vi "Hardware-DIScope.vi"(11 "DSI Reference":refnum<class "DCM-DSI.lvclass">) -> ()   [LabVIEW 2016, in "DSI-RT.lvlib"]
uses:
  DSI-RT.lvlib
  Classes/DCM-DSI/DCM-DSI.lvclass
  <vilib>/Powertrain Controls/Device Drivers/DCM/Rev0/RT/DI - ADC Select.ctl
  <vilib>/Powertrain Controls/Device Drivers/DCM/Rev0/FPGA/DI - ADC Signals.ctl
  <vilib>/Powertrain Controls/Device Drivers/DCM/Rev0/RT/DCM - RT.lvclass/DCM - RT.ctl
  <vilib>/Powertrain Controls/Device Drivers/DCM/Rev0/RT/Read Stop Target.vi
  Classes/DCM-DSI/Read DCM Ref.vi
  Classes/DCM-DSI/Write DI Scope dt.vi
  Classes/DCM-DSI/Write DI Scope Data.vi
  <vilib>/Powertrain Controls/Device Drivers/DCM/Rev0/RT/DCM - RT.lvclass
  <vilib>/addons/Software Calibration Management/xSCM/CalPoint.xnode
  <vilib>/Powertrain Controls/Device Drivers/DCM/DI/RT/DCM - RT - DI.lvlib
  <vilib>/Powertrain Controls/Device Drivers/DCM/Rev0/FPGA/DCM - FPGA.lvlib
  <vilib>/addons/Software Calibration Management/xSCM/ni_scm.dll
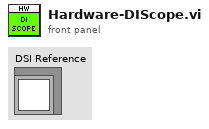
[diagram p1: front panel]
types:
  T1 = typedef "DCM - RT.lvclass/DI - ADC Select.ctl" = cluster{"DI ADC 1":T2, "DI ADC 2":T2, "DI ADC 3":T2, "DI ADC 4":T2}
  T2 = typedef "DCM - FPGA.lvlib/DI - ADC Signals.ctl" = enum8{"I LS A1/A5", "I LS A2/A6", "I LS A3/A7", "I LS A4", "I LS A8/PumpA", "V PZ A1", "V PZ A2", "V PZ A3", "V PZ A4", "V S A1", "V S A2", "V S A3", "V S A4", "V S A5", "V S A6", "V S A7", "V S A8", "V Pump A", "V Secondary A1A2", "V Secondary A3A4", "V Ext HV A", "------------------------ ", "I LS B1/B5", "I LS B2/B6", "I LS B3/B7", "I LS B4", "I LS B8/PumpB", "V PZ B1", "V PZ B2", "V PZ B3", "V PZ B4", "V S B1", "V S B2", "V S B3", "V S B4", "V S B5", "V S B6", "V S B7", "V S B8", "V Pump B", "V Secondary B1B2", "V Secondary B3B4", "V Ext HV B", "-------------------------  ", "AI 1", "AI 2", "AI 3", "AI 4", "AI 5", "AI 6", "AI 7", "AI 8", "AI 9", "AI 10", "AI 11", "AI 12", "-------------------------   ", "V DRVP"}
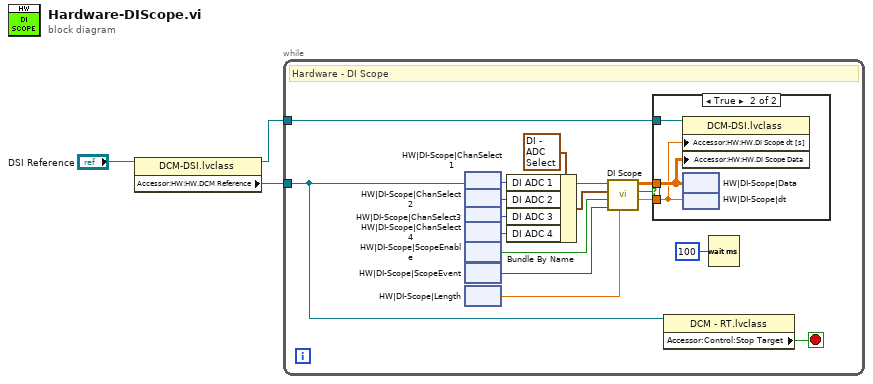
[diagram p0: block diagram]
diagram:
  n1 = property class="DCM-DSI.lvclass"(reference="DSI Reference") -> (reference out=w1:refnum<class "DCM-DSI.lvclass">, "Accessor:HW:HW.DCM Reference"=w2:refnum<class "DCM - RT.lvclass">)  [unwired: 1 in, 1 out]
  n2 = while {
    tunnel: w2 -> [w11]
    tunnel: w1 -> [w6]
    stop <- w10 stop-if-true
    # "Hardware - DI Scope"
    n3 = xnode "HW|DI-Scope|ChanSelect1"() -> ("Value"=w16:u8)
    n4 = xnode "HW|DI-Scope|ChanSelect2"() -> ("Value"=w17:u8)
    n5 = xnode "HW|DI-Scope|ChanSelect3"() -> ("Value"=w13:u8)
    n6 = xnode "HW|DI-Scope|ChanSelect4"() -> ("Value"=w12:u8)
    n7 = xnode "HW|DI-Scope|ScopeEnable"() -> ("Value"=w15:bool)
    n8 = xnode "HW|DI-Scope|ScopeEvent"() -> ("Value"=w14:u8)
    n9 = xnode "HW|DI-Scope|Length"() -> ("Value"=w4:sgl)
    n10 = Bundle By Name(cluster=T1 {"DI ADC 1"=enum."I LS A1/A5", "DI ADC 2"=enum."I LS A1/A5", "DI ADC 3"=enum."I LS A1/A5", "DI ADC 4"=enum."I LS A1/A5"} ("DI ADC Select"), "DI ADC 1"=w16, "DI ADC 2"=w17, "DI ADC 3"=w13, "DI ADC 4"=w12) -> (w19:T1)
    n11 = call <vilib>:"DI Scope.vi"("DI Scope Length [s]"=w4, "DI Scope Event"=w14, "DI Scope Capture"=w15, "Channel Select"=w19, "DCM Reference"=w11) -> ("dT [s]"=w7:sgl, "New Data"=w8:bool, "Data"=w9:sgl[][])  [unwired: 3 in, 1 out]
    n12 = case shown="True" w8 {
      tunnel: w9 -> [_ w56]
      tunnel: w6 -> [_ w57]
      tunnel: w7 -> [_ w55]
      frame False {
      }
      frame True {
        n13 = property class="DCM-DSI.lvclass"(reference=w57, "Accessor:HW:HW.DI Scope dt [s]"=w55, "Accessor:HW:HW.DI Scope Data"=w56) -> ()  [unwired: 1 in, 2 out]
        n14 = xnode "HW|DI-Scope|Data"("Value"=w56) -> ()
        n15 = xnode "HW|DI-Scope|dt"("Value"=w55) -> ()
      }
    }
    n16 = property class="DCM - RT.lvclass"(reference=w11) -> ("Accessor:Control:Stop Target"=w10:bool)  [unwired: 1 in, 2 out]
    n17 = Wait (ms)(milliseconds to wait=u32 100) -> ()  [unwired: 1 out]
  }
